vi "WhileLoop Terminals Info.vi"(8 "error in":errorcluster, 11 "reference":refnum<vi>) -> (0 "error out":errorcluster, 2 "Terminals[]":refnum<vi>[](array[refnum]), 3 "output cluster":T1)   [LabVIEW 2014]
doc: "Convert string ClassName into specific reference ie. Terminal owner which will be SubVI converts this VI to ref.to SubVI so we caqn easily create property and ivnoke methods."
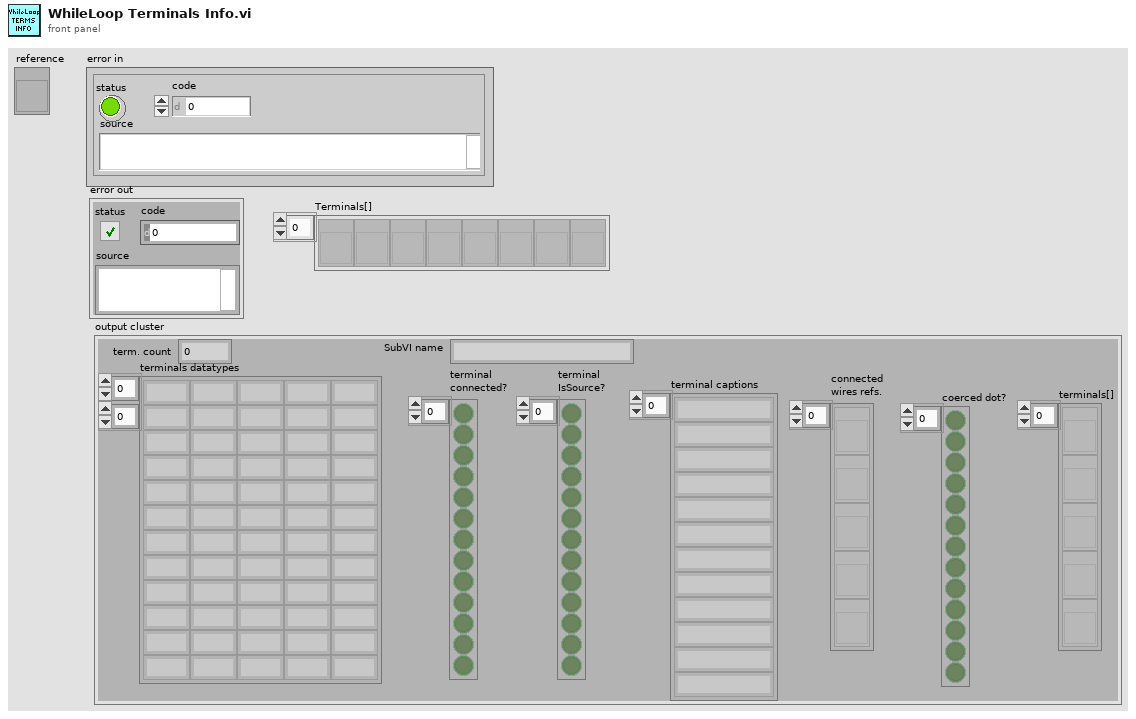
[diagram p1: front panel]
types:
  T1 = cluster{"terminals datatypes":string[][], "terminal\nconnected?":bool[], "terminal captions":string[], "term. count":i32, "terminal\nIsSource?":bool[], "SubVI name":string, "connected\nwires refs.":refnum<vi>[], "coerced dot?":bool[], "terminals[]":refnum<vi>[]}
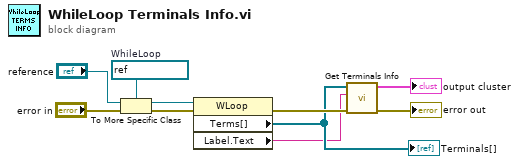
[diagram p0: block diagram]
diagram:
  w10 = refnum<vi> refnum  # WhileLoop
  n1 = To More Specific Class(target class=w10, reference="reference", error in="error in") -> (specific class reference=w8:refnum<vi>, error out=w7:errorcluster)
  n2 = property class="WLoop"(reference=w8, error in=w7) -> (error out=w5:errorcluster, "Terms[]"=w4:refnum<vi>[], "Label.Text"=w1:string)  [unwired: 1 out]
  "Terminals[]" <- w4
  n3 = call "Get Terminals Info.vi"("error in (no error)"=w5, "structure name"=w1, "Terms[]"=w4) -> ("error out"=→"error out":errorcluster, "output cluster"=→"output cluster":T1)  [unwired: 7 in]
